vi "CloseTrig.vi"(8 "error in (no error)":errorcluster, 10 "TrigName":string, 11 "PXI_MultiTrig in":refnum<class "PXI_MultiTrig.lvclass">) -> (0 "error out":errorcluster, 3 "PXI_MultiTrig out":refnum<class "PXI_MultiTrig.lvclass">)   [LabVIEW 2018, in "SyncPlugins.lvlib" / "PXI_MultiTrig.lvclass"]
uses:
  PXI_MultiTrig.lvclass
  PXI_MultiTrig.lvclass/PXI_MultiTrig.ctl
  Accessors/Write Triggers.vi
  Accessors/Read TimingSession.vi
  Accessors/Read RefClkSession.vi
  Accessors/Read Triggers.vi
  <vilib>/Utility/error.llb/Error Cluster From Error Code.vi
  <vilib>/ErrorRing/Error Ring.xnode
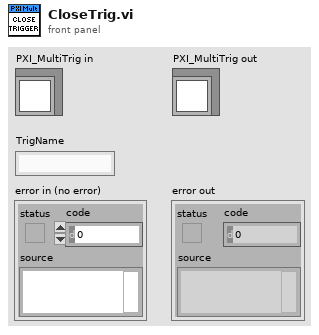
[diagram p1: front panel]
types:
  T1 = typedef "SyncPlugins.lvlib/PXI_MultiTrig.lvclass/clTrigger.ctl" = cluster{"Name":string, "DestTerm":string, "SrcTerm":string, "SyncClk":string, "Edge":i32, "Invert?":i32, "Initiated":bool, "Type":string, "TrigTime":bool}
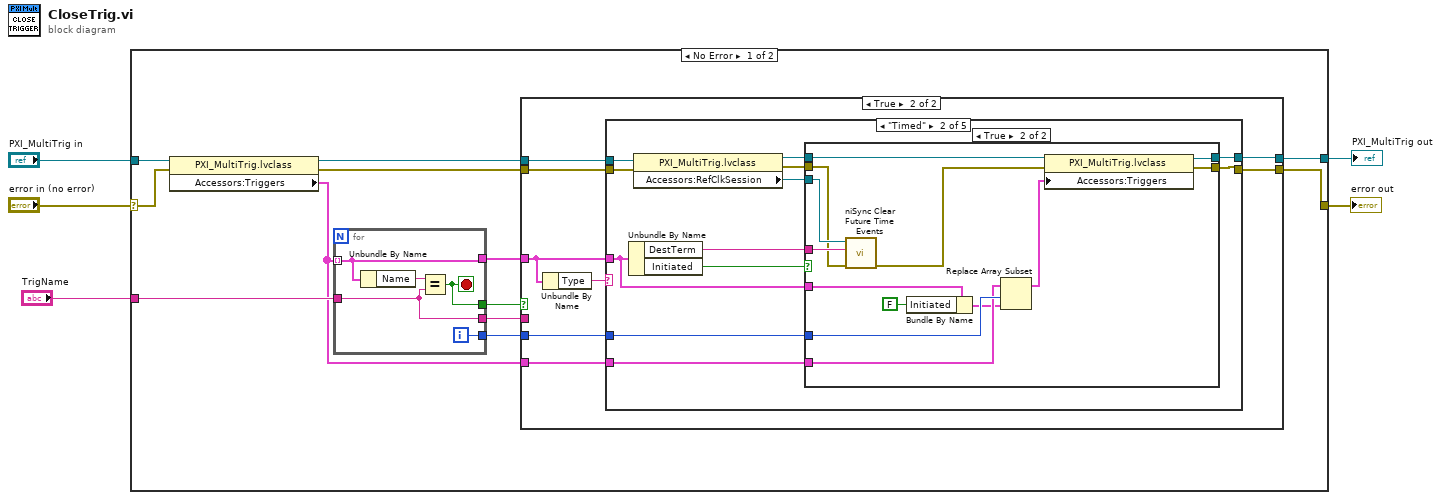
[diagram p0: block diagram]
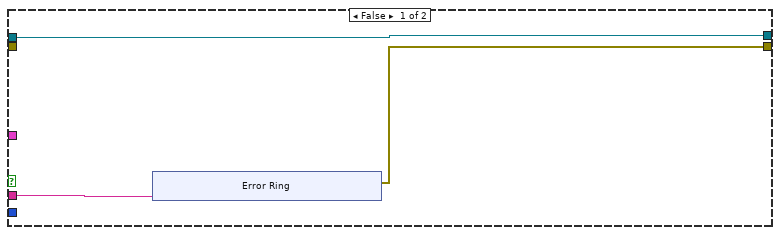
[diagram p2: hidden frame]
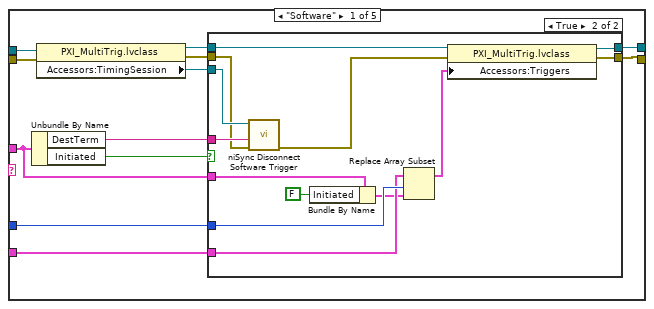
[diagram p3: hidden frame]
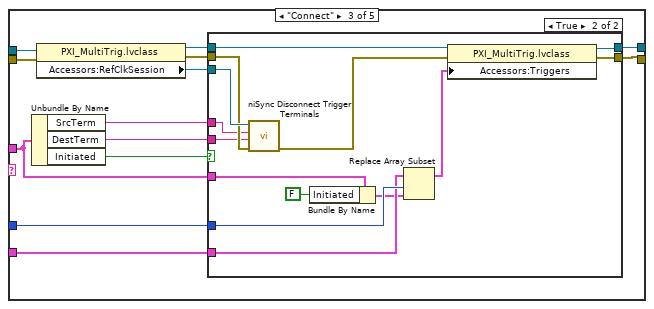
[diagram p6: hidden frame]
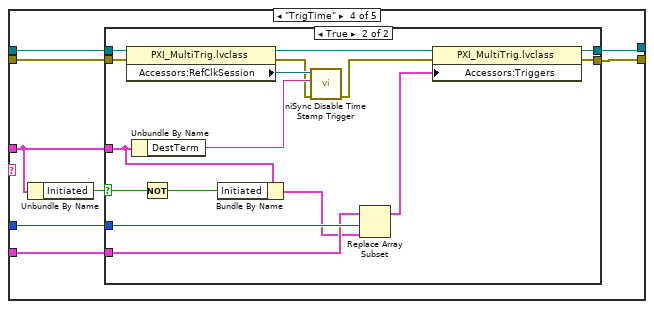
[diagram p8: hidden frame]
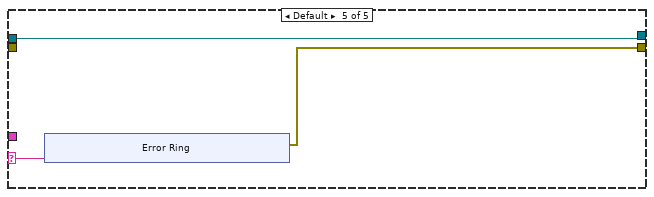
[diagram p10: hidden frame]
diagram:
  n1 = case shown="No Error" "error in (no error)" {
    selector: "error in (no error)" -> [w16 w160]
    tunnel: "PXI_MultiTrig in" -> [w17 w161]
    tunnel: "TrigName" -> [w15 _]
    tunnel: [w8 w161] -> w2
    tunnel: [w7 w160] -> w1
    frame No Error {
      n2 = property class="PXI_MultiTrig.lvclass"(reference=w17, error in=w16) -> (reference out=w12:refnum<class "PXI_MultiTrig.lvclass">, error out=w13:errorcluster, "Accessors:Triggers"=w6:T1[])
      n3 = for {
        tunnel: w6 -> [w158] mode=indexing
        tunnel: w15 -> [w156]
        tunnel: [w158] -> w11
        tunnel: [w157] -> w14
        tunnel: [w156] -> w10
        tunnel: [w155] -> w9
        i -> [w155]
        stop <- w157 stop-if-true
        n4 = Unbundle By Name(w158) -> ("Name"=w159:string)
        n5 = Equal?(x=w159, y=w156) -> (x = y?=w157:bool)
      }
      n6 = case shown="True" w14 {
        tunnel: w13 -> [_ w32]
        tunnel: w12 -> [w19 w33]
        tunnel: w11 -> [_ w31]
        tunnel: w10 -> [w20 _]
        tunnel: w9 -> [_ w28]
        tunnel: [w19 w30] -> w8
        tunnel: [w18 w34] -> w7
        tunnel: w6 -> [_ w29]
        frame False {
          n7 = xnode "Error Ring"("parameter 0"=w20) -> ("error out"=w18:errorcluster)
        }
        frame True {
          n8 = Unbundle By Name(w31) -> ("Type"=w35:string)
          n9 = case shown="\"Timed\"" w35 {
            selector: w35 -> [_ _ _ _ w147]
            tunnel: [w39 w66 w94 w121 w146] -> w34
            tunnel: w33 -> [w47 w74 w102 w123 w145]
            tunnel: w32 -> [w46 w73 w101 w124 _]
            tunnel: w31 -> [w37 w64 w92 w125 _]
            tunnel: [w40 w67 w95 w122 w145] -> w30
            tunnel: w29 -> [w38 w65 w93 w120 _]
            tunnel: w28 -> [w36 w63 w91 w119 _]
            frame "Software" {
              n10 = Unbundle By Name(w37) -> ("DestTerm"=w41:string, "Initiated"=w42:bool)
              n11 = property class="PXI_MultiTrig.lvclass"(reference=w47, error in=w46) -> (reference out=w45:refnum<class "PXI_MultiTrig.lvclass">, error out=w44:errorcluster, "Accessors:TimingSession"=w43:refnum<k15>)
              n12 = case shown="True" w42 {
                tunnel: w45 -> [w49 w52]
                tunnel: w44 -> [w48 w60]
                tunnel: w43 -> [_ w61]
                tunnel: w41 -> [_ w62]
                tunnel: [w49 w53] -> w40
                tunnel: [w48 w54] -> w39
                tunnel: w38 -> [_ w56]
                tunnel: w37 -> [_ w58]
                tunnel: w36 -> [_ w57]
                frame False {
                }
                frame True {
                  n13 = call <instrlib>:"niSync Disconnect Software Trigger.vi"("error in (no error)"=w60, "destination terminal"=w62, "instrument handle"=w61) -> ("error out"=w50:errorcluster)  [unwired: 7 in, 1 out]
                  n14 = Bundle By Name(cluster=w58, "Initiated"=FALSE) -> (w55:T1)
                  n15 = Replace Array Subset(array=w56, new element=w55, index=w57) -> (w51:T1[])
                  n16 = property class="PXI_MultiTrig.lvclass"(reference=w52, error in=w50, "Accessors:Triggers"=w51) -> (reference out=w53:refnum<class "PXI_MultiTrig.lvclass">, error out=w54:errorcluster)
                }
              }
            }
            frame "Timed" {
              n17 = Unbundle By Name(w64) -> ("DestTerm"=w68:string, "Initiated"=w69:bool)
              n18 = property class="PXI_MultiTrig.lvclass"(reference=w74, error in=w73) -> (reference out=w72:refnum<class "PXI_MultiTrig.lvclass">, error out=w71:errorcluster, "Accessors:RefClkSession"=w70:refnum<k15>)
              n19 = case shown="True" w69 {
                tunnel: w72 -> [w76 w79]
                tunnel: w71 -> [w75 w87]
                tunnel: w70 -> [_ w88]
                tunnel: w68 -> [_ w89]
                tunnel: [w76 w80] -> w67
                tunnel: [w75 w81] -> w66
                tunnel: w65 -> [_ w83]
                tunnel: w64 -> [_ w85]
                tunnel: w63 -> [_ w84]
                frame False {
                }
                frame True {
                  n20 = call <instrlib>:"niSync Clear Future Time Events.vi"("error in (no error)"=w87, "terminal"=w89, "instrument handle"=w88) -> ("error out"=w77:errorcluster)  [unwired: 6 in, 1 out]
                  n21 = Bundle By Name(cluster=w85, "Initiated"=FALSE) -> (w82:T1)
                  n22 = Replace Array Subset(array=w83, new element=w82, index=w84) -> (w78:T1[])
                  n23 = property class="PXI_MultiTrig.lvclass"(reference=w79, error in=w77, "Accessors:Triggers"=w78) -> (reference out=w80:refnum<class "PXI_MultiTrig.lvclass">, error out=w81:errorcluster)
                }
              }
            }
            frame "Connect" {
              n24 = Unbundle By Name(w92) -> ("SrcTerm"=w90:string, "DestTerm"=w96:string, "Initiated"=w97:bool)
              n25 = property class="PXI_MultiTrig.lvclass"(reference=w102, error in=w101) -> (reference out=w100:refnum<class "PXI_MultiTrig.lvclass">, error out=w99:errorcluster, "Accessors:RefClkSession"=w98:refnum<k15>)
              n26 = case shown="True" w97 {
                tunnel: w100 -> [w104 w109]
                tunnel: w99 -> [w103 w117]
                tunnel: w98 -> [_ w118]
                tunnel: w96 -> [_ w106]
                tunnel: [w104 w110] -> w95
                tunnel: [w103 w111] -> w94
                tunnel: w93 -> [_ w113]
                tunnel: w92 -> [_ w115]
                tunnel: w91 -> [_ w114]
                tunnel: w90 -> [_ w105]
                frame False {
                }
                frame True {
                  n27 = call <instrlib>:"niSync Disconnect Trigger Terminals.vi"("error in (no error)"=w117, "destination terminal"=w106, "source terminal"=w105, "instrument handle"=w118) -> ("error out"=w107:errorcluster)  [unwired: 6 in, 1 out]
                  n28 = Bundle By Name(cluster=w115, "Initiated"=FALSE) -> (w112:T1)
                  n29 = Replace Array Subset(array=w113, new element=w112, index=w114) -> (w108:T1[])
                  n30 = property class="PXI_MultiTrig.lvclass"(reference=w109, error in=w107, "Accessors:Triggers"=w108) -> (reference out=w110:refnum<class "PXI_MultiTrig.lvclass">, error out=w111:errorcluster)
                }
              }
            }
            frame "TrigTime" {
              n31 = Unbundle By Name(w125) -> ("Initiated"=w126:bool)
              n32 = case shown="True" w126 {
                selector: w126 -> [_ w139]
                tunnel: w125 -> [_ w138]
                tunnel: w124 -> [w127 w143]
                tunnel: w123 -> [w128 w144]
                tunnel: [w128 w130] -> w122
                tunnel: [w127 w129] -> w121
                tunnel: w120 -> [_ w135]
                tunnel: w119 -> [_ w136]
                frame False {
                }
                frame True {
                  n33 = property class="PXI_MultiTrig.lvclass"(reference=w144, error in=w143) -> (reference out=w133:refnum<class "PXI_MultiTrig.lvclass">, error out=w140:errorcluster, "Accessors:RefClkSession"=w142:refnum<k15>)
                  n34 = Unbundle By Name(w138) -> ("DestTerm"=w141:string)
                  n35 = Not(x=w139) -> (.not. x?=w137:bool)
                  n36 = Bundle By Name(cluster=w138, "Initiated"=w137) -> (w134:T1)
                  n37 = call <instrlib>:"niSync Disable Time Stamp Trigger.vi"("error in (no error)"=w140, "terminal"=w141, "instrument handle"=w142) -> ("error out"=w132:errorcluster)  [unwired: 6 in, 1 out]
                  n38 = Replace Array Subset(array=w135, new element=w134, index=w136) -> (w131:T1[])
                  n39 = property class="PXI_MultiTrig.lvclass"(reference=w133, error in=w132, "Accessors:Triggers"=w131) -> (reference out=w130:refnum<class "PXI_MultiTrig.lvclass">, error out=w129:errorcluster)
                }
              }
            }
            frame Default {
              n40 = xnode "Error Ring"("parameter 0"=w147) -> ("error out"=w146:errorcluster)
            }
          }
        }
      }
    }
    frame Error {
    }
  }
  "error out" <- w1
  "PXI_MultiTrig out" <- w2
